vi "target.vi"   [LabVIEW 2020]
uses:
  <vilib>/rvi/interface/RandomDataEmulation/niFpgaRandomDataHandleErrors.vi
  <vilib>/rvi/DataTransferAndStorage/Container/XNode/niFpgaContainer.xnode
  <vilib>/rvi/interface/RandomDataEmulation/nirviRandomDataFpgaReadWriteTemplate.vi
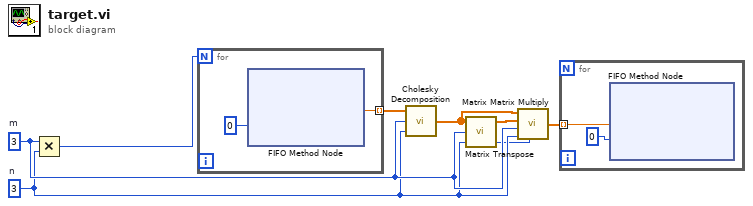
[diagram p0: block diagram]
diagram:
  w5 = 3  # n
  w6 = 3  # m
  n1 = Multiply(x=w6, y=w5) -> (x*y=w8:i32)
  n2 = for {
    N: w8 -> [_]
    tunnel: [w10] -> w7 mode=indexing
    n3 = xnode ("FIFO Method Node")("Timeout"=0) -> ("Element"=w10:sgl)  [unwired: 1 in, 2 out]
  }
  n4 = call <vilib>:"Cholesky Decomposition.vi"("n"=w5, "m"=w6, "A"=w7) -> ("L"=w3:sgl[])
  n5 = call <vilib>:"Matrix Transpose.vi"("n"=w5, "m"=w6, "A"=w3) -> ("n"=w1:i32, "B"=w2:sgl[])  [unwired: 1 out]
  n6 = call <vilib>:"Matrix Matrix Multiply.vi"("p"=w1, "n"=w5, "m"=w6, "B"=w2, "A"=w3) -> ("C"=w4:sgl[])  [unwired: 1 in]
  n7 = for {
    tunnel: w4 -> [w11] mode=indexing
    n8 = xnode ("FIFO Method Node")("Element"=w11, "Timeout"=0) -> ()  [unwired: 1 in, 2 out]
  }
